vi "Determine Array and Scrollbar Properties.vi"(8 "error in":errorcluster, 10 "Coords of Click":T1, 11 "Array Reference":refnum<vi>) -> (0 "error out":errorcluster, 1 "Scrollbar Properties":T2, 2 "Array Properties":T5, 3 "dup Array Reference":refnum<vi>)   [LabVIEW 2020, in "Determine Clicked Array Element Index.lvlib"]
doc: "Determine Clicked Array Element Index - Determine Array and Scrollbar Properties.vi\n\nDescription:\nThis VI determines multiple properties of the array and scrollbars of the array specified by the Array Reference input.\n\nIf no caption has been created for the array of interest, instruct the user how to correct the issue.\n\nInputs:\nArray Reference - Reference to the array to operate on.\n\nCoords of Click - The screen coordinates of the click within the array. These values are used to determine if the click occurred on the selected item.\n\nerror in - Standard error cluster.\n\nOutputs:\ndup Array Reference - Dup reference to the array to operate on.\n\nArray Properties - Cluster containing the array properties of the array specified by the Array Reference input.\n\nScrollbar Properties - Cluster containing the scrollbar properties of the array specified by the Array Reference input.\n\nerror out - standard error cluster.\n\nDeveloped By:\nMark.ridgley\nMark.Ridgley_LabVIEW.Developer@comcast.net"
uses:
  Determine Clicked Array Element Index.lvlib
  <vilib>/Utility/miscctls.llb/LVPositionTypeDef.ctl
  <vilib>/Utility/miscctls.llb/LVBoundsTypeDef.ctl
  <vilib>/Utility/miscctls.llb/LVPoint32TypeDef.ctl
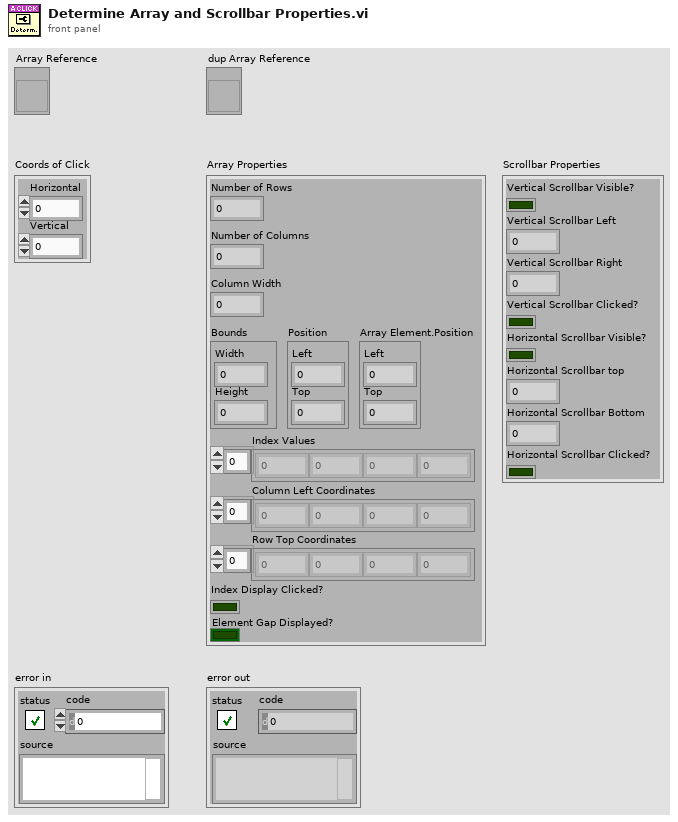
[diagram p1: front panel]
types:
  T1 = typedef "LVPoint32TypeDef.ctl" = cluster{"Horizontal":i32, "Vertical":i32}
  T2 = cluster{"Vertical Scrollbar Visible?":bool, "Vertical Scrollbar Left":i32, "Vertical Scrollbar Right":i32, "Vertical Scrollbar Clicked?":bool, "Horizontal Scrollbar Visible? ":bool, "Horizontal Scrollbar top":i32, "Horizontal Scrollbar Bottom":i32, "Horizontal Scrollbar Clicked?":bool}
  T3 = typedef "LVBoundsTypeDef.ctl" = cluster{"Width":u32, "Height":u32}
  T4 = typedef "LVPositionTypeDef.ctl" = cluster{"Left":i32, "Top":i32}
  T5 = cluster{"Number of Rows":u32, "Number of Columns":u32, "Column Width":u32, "Bounds":T3, "Position":T4, "Array Element.Position":T4, "Index Values":u32[], "Column Left Coordinates":i32[], "Row Top Coordinates":i32[], "Index Display Clicked?":bool, "Element Gap Displayed?":bool}
  T6 = enum16{"Horizontal Scrollbar", "Vertical Scrollbar"}
  T7 = enum16{"Horizontal Scrollbar", "Vertical Scrollbar", "Index Display"}
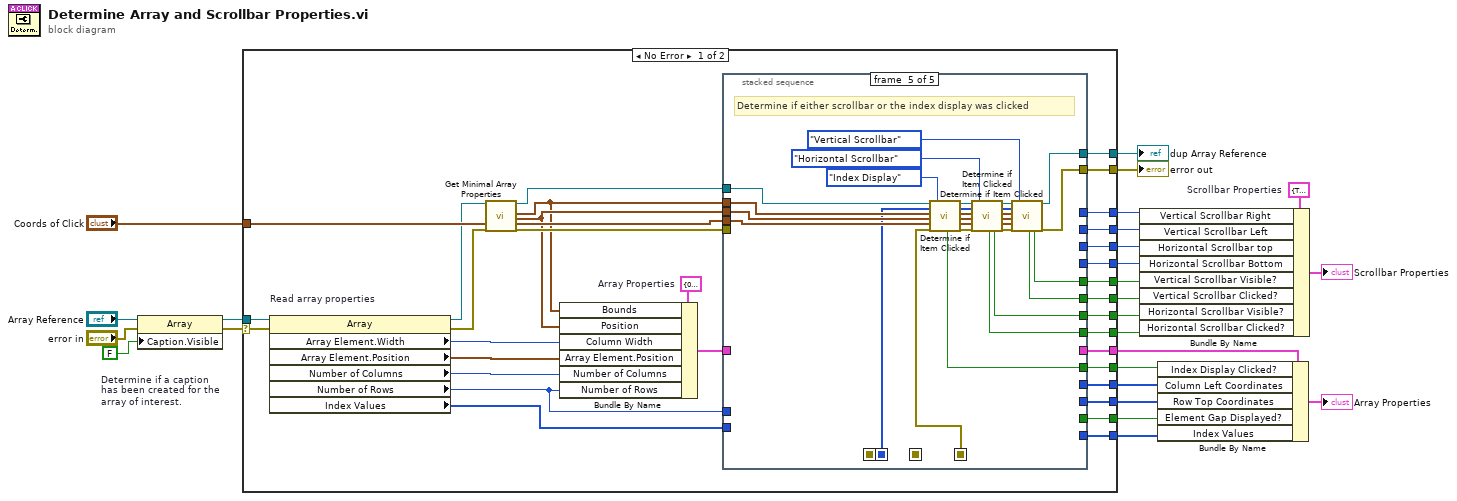
[diagram p0: block diagram]
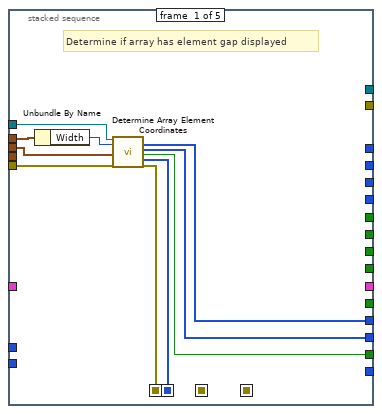
[diagram p2: hidden frame]
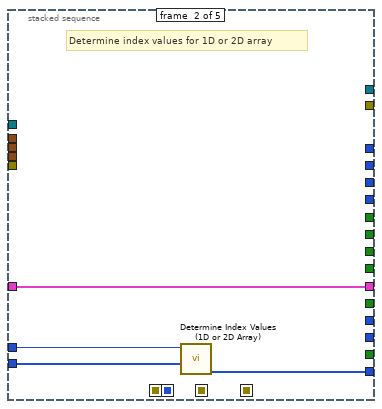
[diagram p3: hidden frame]
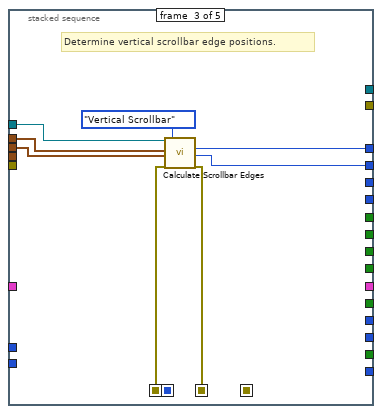
[diagram p4: hidden frame]
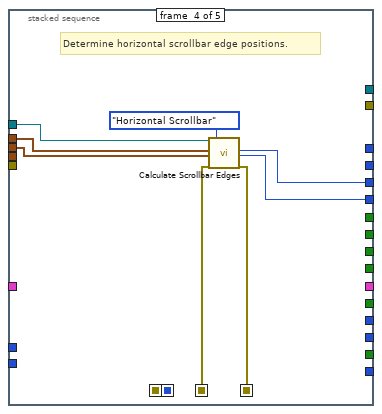
[diagram p5: hidden frame]
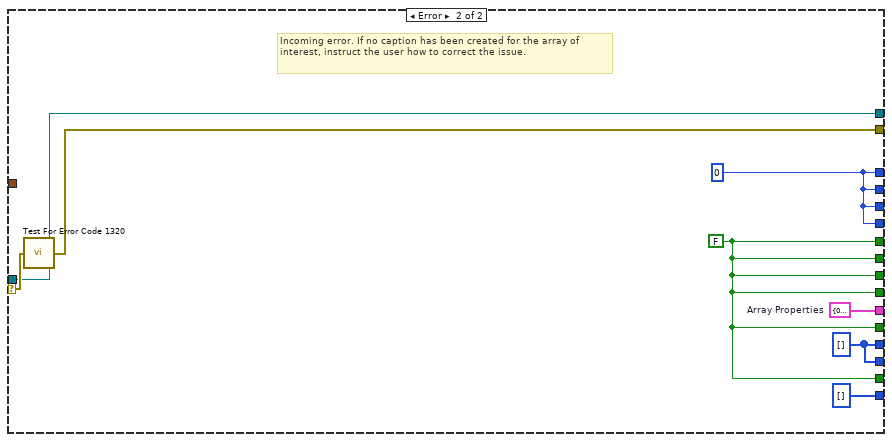
[diagram p6: hidden frame]
diagram:
  w1 = T2 {"Vertical Scrollbar Visible?"=TRUE, "Vertical Scrollbar Left"=0, "Vertical Scrollbar Right"=0, "Vertical Scrollbar Clicked?"=FALSE, "Horizontal Scrollbar Visible? "=TRUE, "Horizontal Scrollbar top"=0, "Horizontal Scrollbar Bottom"=0, "Horizontal Scrollbar Clicked?"=TRUE}  # Scrollbar Properties
  n1 = property on="Determine if a caption has been created for the array of interest." class="Array"(reference="Array Reference", error in="error in", "Caption.Visible"=FALSE) -> (reference out=w6:refnum<vi>, error out=w23:errorcluster)
  n2 = case shown="No Error" w23 {
    selector: w23 -> [w55 w124]
    tunnel: "Coords of Click" -> [w54 _]
    tunnel: [w53 u32[] [] ("Column Left Coordinates")] -> w20
    tunnel: w6 -> [w52 w122]
    tunnel: [w50 w121] -> w19
    tunnel: [w49 w121] -> w18
    tunnel: [w48 w121] -> w17
    tunnel: [w47 w121] -> w16
    tunnel: [w46 w121] -> w15
    tunnel: [w44 w122] -> w14
    tunnel: [w43 w117] -> w13
    tunnel: [w42 w117] -> w12
    tunnel: [w40 w120] -> w11
    tunnel: [w39 w120] -> w10
    tunnel: [w38 w121] -> w9
    tunnel: [w30 w118] -> w8
    tunnel: [w56 w123] -> w25
    tunnel: [w27 w117] -> w3
    tunnel: [w26 w117] -> w2
    frame No Error {
      w28 = T5 {"Number of Rows"=0, "Number of Columns"=0, "Column Width"=0, "Bounds"={"Width"=0, "Height"=0}, "Position"={"Left"=0, "Top"=0}, "Array Element.Position"={"Left"=0, "Top"=0}, "Index Values"=[], "Column Left Coordinates"=[], "Row Top Coordinates"=[], "Index Display Clicked?"=FALSE, "Element Gap Displayed?"=FALSE}  # Array Properties
      n3 = property on="Read array properties" class="Array"(reference=w52, error in=w55) -> (reference out=w51:refnum<vi>, error out=w58:errorcluster, "Array Element.Width"=w29:u32, "Array Element.Position"=w34:T4, "Number of Columns"=w32:u32, "Number of Rows"=w33:u32, "Index Values"=w35:u32[])
      n4 = call "Get Minimal Array Properties.vi"("Array Reference"=w51, "Coords of Click"=w54, "error in"=w58) -> ("dup Array Reference"=w41:refnum<vi>, "Minimal Array Properties.Bounds"=w36:T3, "Minimal Array Properties.Position"=w37:T4, "dup Coords of Click"=w45:T1, "error out"=w57:errorcluster)  [unwired: 12 in]
      n5 = Bundle By Name(cluster=w28, "Bounds"=w36, "Position"=w37, "Column Width"=w29, "Array Element.Position"=w34, "Number of Columns"=w32, "Number of Rows"=w33) -> (w31:T5)
      n6 = stacked-sequence {
        seq-local: [w62 _ _ _ _] -> [_ _ _ _ w90]
        seq-local: [w67 _ _ _ _] -> [_ _ w80 _ _]
        seq-local: [_ _ w79 _ _] -> [_ _ _ w88 _]
        seq-local: [_ _ _ w87 _] -> [_ _ _ _ w113]
        tunnel: [_ w69 _ _ _] -> w53
        tunnel: w35 -> [_ w72 _ _ _]
        tunnel: [_ _ _ _ w110] -> w50
        tunnel: [_ _ _ _ w109] -> w49
        tunnel: [_ _ _ _ w108] -> w48
        tunnel: [_ _ _ _ w107] -> w47
        tunnel: [_ _ _ _ w106] -> w46
        tunnel: w45 -> [_ _ _ _ w94]
        tunnel: w57 -> [w68 _ _ _ _]
        tunnel: [_ _ _ _ w89] -> w44
        tunnel: [_ _ _ _ w114] -> w56
        tunnel: [_ _ w77 _ _] -> w43
        tunnel: [_ _ w76 _ _] -> w42
        tunnel: w36 -> [w60 _ w75 w83 w93]
        tunnel: w33 -> [_ w71 _ _ _]
        tunnel: w37 -> [w61 _ w74 w82 w92]
        tunnel: w41 -> [w66 _ w78 w86 w91]
        tunnel: [w65 _ _ _ _] -> w40
        tunnel: [w64 _ _ _ _] -> w39
        tunnel: [w63 _ _ _ _] -> w38
        tunnel: w31 -> [_ w70 _ _ _]
        tunnel: [_ w70 _ _ _] -> w30
        tunnel: [_ _ _ w85 _] -> w27
        tunnel: [_ _ _ w84 _] -> w26
        frame #0 {
          # "Determine if array has element gap displayed"
          n7 = Unbundle By Name(w60) -> ("Width"=w59:u32)
          n8 = call "Determine Array Element Coordinates.vi"("Array Reference"=w66, "Minimal Array Properties.Bounds.Width"=w59, "Minimal Array Properties.Position"=w61, "error in"=w68) -> ("Column Left Coordinates"=w65:i32[], "Row Top Coordinates"=w64:i32[], "Array has element gap?"=w63:bool, "Un-gapped left coordinates"=w62:i32[], "error out"=w67:errorcluster)  [unwired: 10 in, 1 out]
        }
        frame #1 {
          # "Determine index values for 1D or 2D array"
          n9 = call "Determine Index Values (1D or 2D Array).vi"("Array Property.Index Values"=w72, "Array Property.Number of Rows"=w71) -> ("Index Values (1D or 2D Array)"=w69:u32[])  [unwired: 9 in]
        }
        frame #2 {
          # "Determine vertical scrollbar edge positions."
          n10 = call "Calculate Scrollbar Edges.vi"("Array Reference"=w78, "Minimal Array Properties.Bounds"=w75, "Minimal Array Properties.Position"=w74, "error in (no error)"=w80, "Select Item"=T6."Vertical Scrollbar") -> ("Minimum Scrollbar Edge"=w76:i32, "Maximum Scrollbar Edge"=w77:i32, "error out"=w79:errorcluster)  [unwired: 11 in, 1 out]
        }
        frame #3 {
          # "Determine horizontal scrollbar edge positions."
          n11 = call "Calculate Scrollbar Edges.vi"("Array Reference"=w86, "Minimal Array Properties.Bounds"=w83, "Minimal Array Properties.Position"=w82, "error in (no error)"=w88, "Select Item"=T6."Horizontal Scrollbar") -> ("Minimum Scrollbar Edge"=w85:i32, "Maximum Scrollbar Edge"=w84:i32, "error out"=w87:errorcluster)  [unwired: 11 in, 1 out]
        }
        frame #4 {
          # "Determine if either scrollbar or the index display was clicked"
          n12 = call "Determine if Item Clicked.vi"("Array Reference"=w91, "Un-gapped left coordinates"=w90, "Minimal Array Properties.Bounds"=w93, "Minimal Array Properties.Position"=w92, "Coords of Click"=w94, "error in"=w113, "Select Item"=T7."Index Display") -> ("Item Clicked?"=w110:bool, "dup Array Reference"=w112:refnum<vi>, "dup Un-gapped left coordinates"=w99:i32[], "dup Minimal Array Properties.Bounds"=w105:T3, "dup Minimal Array Properties.Position"=w101:T4, "dup Coords of Click"=w100:T1, "error out"=w115:errorcluster)  [unwired: 5 in, 1 out]
          n13 = call "Determine if Item Clicked.vi"("Array Reference"=w112, "Un-gapped left coordinates"=w99, "Minimal Array Properties.Bounds"=w105, "Minimal Array Properties.Position"=w101, "Coords of Click"=w100, "error in"=w115, "Select Item"=T7."Horizontal Scrollbar") -> ("Item Clicked?"=w109:bool, "Item Visible?"=w108:bool, "dup Array Reference"=w111:refnum<vi>, "dup Un-gapped left coordinates"=w98:i32[], "dup Minimal Array Properties.Bounds"=w104:T3, "dup Minimal Array Properties.Position"=w103:T4, "dup Coords of Click"=w102:T1, "error out"=w116:errorcluster)  [unwired: 5 in]
          n14 = call "Determine if Item Clicked.vi"("Array Reference"=w111, "Un-gapped left coordinates"=w98, "Minimal Array Properties.Bounds"=w104, "Minimal Array Properties.Position"=w103, "Coords of Click"=w102, "error in"=w116, "Select Item"=T7."Vertical Scrollbar") -> ("Item Clicked?"=w107:bool, "Item Visible?"=w106:bool, "dup Array Reference"=w89:refnum<vi>, "error out"=w114:errorcluster)  [unwired: 5 in, 4 out]
        }
      }
    }
    frame Error {
      w118 = T5 {"Number of Rows"=0, "Number of Columns"=0, "Column Width"=0, "Bounds"={"Width"=0, "Height"=0}, "Position"={"Left"=0, "Top"=0}, "Array Element.Position"={"Left"=0, "Top"=0}, "Index Values"=[], "Column Left Coordinates"=[], "Row Top Coordinates"=[], "Index Display Clicked?"=FALSE, "Element Gap Displayed?"=FALSE}  # Array Properties
      w120 = i32[] [] ("Column Left Coordinates")
      w117 = 0 ("Vertical Scrollbar Right")
      w121 = FALSE ("Item Visible?")
      # "Incoming error. If no caption has been created for the array of interest, instruct the user how to correct the issue."
      n15 = call "Test For Error Code 1320.vi"("error in"=w124) -> ("error out"=w123:errorcluster)  [unwired: 14 in]
    }
  }
  "error out" <- w25
  "dup Array Reference" <- w14
  n16 = Bundle By Name(cluster=w1, "Vertical Scrollbar Right"=w12, "Vertical Scrollbar Left"=w13, "Horizontal Scrollbar top"=w3, "Horizontal Scrollbar Bottom"=w2, "Vertical Scrollbar Visible?"=w15, "Vertical Scrollbar Clicked?"=w16, "Horizontal Scrollbar Visible?"=w17, "Horizontal Scrollbar Clicked?"=w18) -> (→"Scrollbar Properties":T2)
  n17 = Bundle By Name(cluster=w8, "Index Display Clicked?"=w19, "Column Left Coordinates"=w11, "Row Top Coordinates"=w10, "Element Gap Displayed?"=w9, "Index Values"=w20) -> (→"Array Properties":T5)
